vi "Add Crank Cam RTM.vi"(8 "error in (no error)":errorcluster, 11 "Node Ptr":u64 format="%.0x") -> (0 "error out":errorcluster)   [LabVIEW 2011, in "Engine Sim System Explorer.lvlib"]
uses:
  Engine Sim System Explorer.lvlib
  TypeDefs/NTeethComp.ctl
  TypeDefs/FullyCustomComp.ctl
  Shared/FullyCustomCommMode.ctl
  TypeDefs/FullyCustomProfilesComp.ctl
  <vilib>/NI Veristand/Custom Device API/Custom Device Channel.ctl
  <vilib>/NI Veristand/Custom Device API/Custom Device Channel Type.ctl
  Utility/Add Data Replay.vi
  Shared/Engine Simulation Global.vi
  <vilib>/NI Veristand/Custom Device API/Get Item Property (Variant).vi
  Utility/Set Data Replay Component Properties.vi
  <vilib>/NI Veristand/Custom Device API/NI VeriStand - Set Item Property.vi
  <vilib>/NI Veristand/Custom Device API/Set Item Property (Boolean).vi
  <vilib>/Utility/error.llb/Error Cluster From Error Code.vi
  <vilib>/NI Veristand/Custom Device API/Custom Device API.lvlib
  Engine Simulation Shared.lvlib
  <vilib>/NI Veristand/Custom Device Tools/Custom Device Utility Library/Custom Device Utility Library.lvlib
panel:
  in  "Tag":string
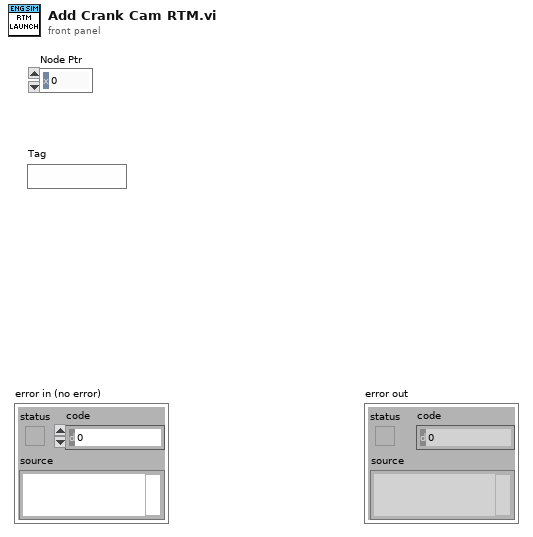
[diagram p1: front panel]
types:
  T1 = typedef "Custom Device API.lvlib/Custom Device Channel.ctl" = cluster{"Type":T2, "Units":string, "Default Value":dbl, "Faultable":bool, "Scalable":bool}
  T2 = typedef "Custom Device API.lvlib/Custom Device Channel Type.ctl" = enum16{"Input", "Output"}
  T3 = typedef "Engine Sim System Explorer.lvlib/FullyCustomComp.ctl" = cluster{"Name":string, "Comm Mode":T4, "Profiles":T5[]}
  T4 = typedef "Engine Simulation Shared.lvlib/FullyCustomCommMode.ctl" = enum16{"DMA FIFO", "FP Data Transfer"}
  T5 = typedef "Engine Sim System Explorer.lvlib/FullyCustomProfilesComp.ctl" = cluster{"Name":string, "Offset?":bool}
  T6 = typedef "Engine Sim System Explorer.lvlib/NTeethComp.ctl" = cluster{"Name":string, "TDC Offset":bool}
  T7 = typedef "Custom Device API.lvlib/Custom Device Item Ref.ctl" = u64
  T8 = typedef "Engine Sim System Explorer.lvlib/DataReplayLoopComp.ctl" = cluster{"Name":string, "DataReplays":T9[]}
  T9 = typedef "Engine Sim System Explorer.lvlib/DataReplayComp.ctl" = cluster{"Name":string, "Number":i32, "Optionals":bool[]}
  T10 = typedef "Custom Device API.lvlib/Custom Device Item Info.ctl" = cluster{"Name":string, "Is Channel":bool, "GUID":string}
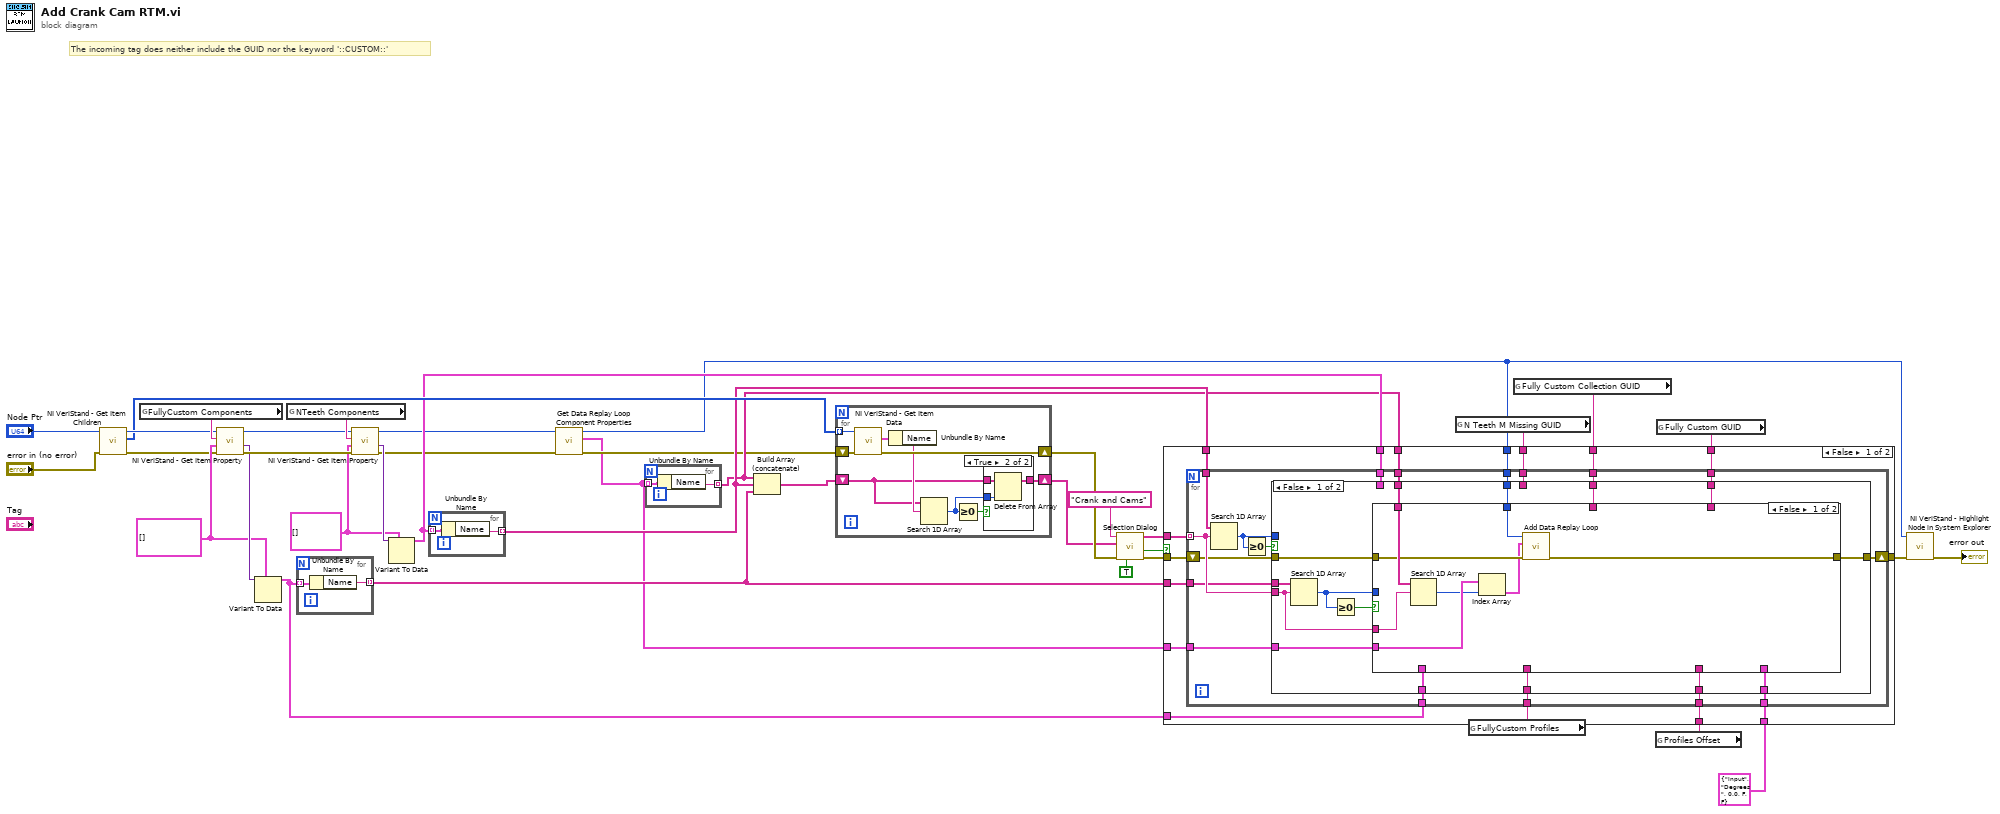
[diagram p0: block diagram]
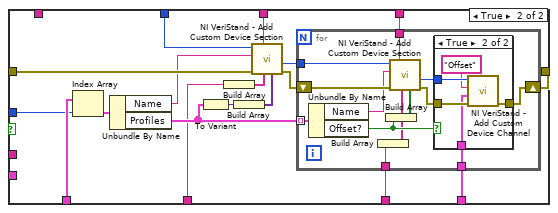
[diagram p2: hidden frame]
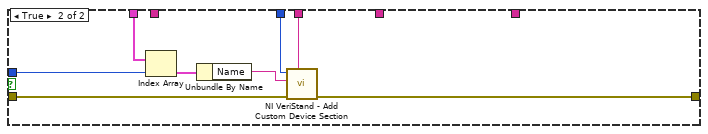
[diagram p4: hidden frame]
diagram:
  w33 = T3[] []
  w31 = T6[] []
  # "The incoming tag does neither include the GUID nor the keyword '::CUSTOM::'"
  n1 = call <vilib>:"NI VeriStand - Get Item Children.vi"("error in (no error)"="error in (no error)", "Item Ref in"="Node Ptr") -> ("error out"=w28:errorcluster, "Child Refs"=w29:T7[], "Item Ref out"=w30:T7)  [unwired: 6 in, 1 out]
  n2 = global read "Engine Simulation Global.vi" "FullyCustom Components"() -> (w38:string)
  n3 = call-poly <vilib>:"NI VeriStand - Get Item Property.vi"("error in (no error)"=w28, "Default Value"=w33, "Property Name"=w38, "Item Ref in"=w30) -> ("error out"=w35:errorcluster, "Value"=w34:variant, "Item Ref out"=w36:T7)  [unwired: 4 in, 1 out]
  n4 = Variant To Data(type=w33, Variant=w34) -> (data=w18:T3[])  [unwired: 1 in, 1 out]
  n5 = global read "Engine Simulation Global.vi" "NTeeth Components"() -> (w37:string)
  n6 = for {
    tunnel: w18 -> [w40] mode=indexing
    tunnel: [w39] -> w19 mode=indexing
    n7 = Unbundle By Name(w40) -> ("Name"=w39:string)
  }
  n8 = call-poly <vilib>:"NI VeriStand - Get Item Property.vi"("error in (no error)"=w35, "Default Value"=w31, "Property Name"=w37, "Item Ref in"=w36) -> ("error out"=w8:errorcluster, "Value"=w32:variant, "Item Ref out"=w7:T7)  [unwired: 4 in, 1 out]
  n9 = Variant To Data(type=w31, Variant=w32) -> (data=w20:T6[])  [unwired: 1 in, 1 out]
  n10 = for {
    tunnel: w20 -> [w42] mode=indexing
    tunnel: [w41] -> w21 mode=indexing
    n11 = Unbundle By Name(w42) -> ("Name"=w41:string)
  }
  n12 = call "Get Data Replay Loop Component Properties.vi"("error in (no error)"=w8, "Item Ref in"=w7) -> ("error out"=w2:errorcluster, "DataReplayLoops"=w1:T8[], "Item Ref out"=w6:T7)  [unwired: 7 in]
  n13 = for {
    tunnel: w1 -> [w44] mode=indexing
    tunnel: [w43] -> w5 mode=indexing
    n14 = Unbundle By Name(w44) -> ("Name"=w43:string)
  }
  n15 = Build Array (concatenate)(w5, w21, w19) -> (w27:string[])
  n16 = for {
    tunnel: w29 -> [w53] mode=indexing
    shift-right: [w51] -> w24
    shift-left: w2 -> [w50]
    shift-right: [w46] -> w3
    shift-left: w27 -> [w47]
    n17 = call <vilib>:"NI VeriStand - Get Item Data.vi"("error in (no error)"=w50, "Item Ref in"=w53) -> ("error out"=w51:errorcluster, "Item Info"=w52:T10)  [unwired: 6 in, 2 out]
    n18 = Unbundle By Name(w52) -> ("Name"=w48:string)
    n19 = Search 1D Array(1D array=w47, element=w48) -> (index of element=w45:i32)  [unwired: 1 in]
    n20 = Greater Or Equal To 0?(x=w45) -> (x >= 0?=w49:bool)
    n21 = case shown="True" w49 {
      tunnel: w47 -> [w54 w57]
      tunnel: [w54 w56] -> w46
      tunnel: w45 -> [_ w55]
      frame False {
      }
      frame True {
        n22 = Delete From Array(array=w57, index=w55) -> (array with subset deleted=w56:string[])  [unwired: 1 in, 1 out]
      }
    }
  }
  n23 = call "Selection Dialog.vi"("Multi-Selection?"=TRUE, "error in (no error)"=w24, "Tree Items"=w3, "Root Tag"="Crank and Cams") -> ("error out"=w22:errorcluster, "Canceled"=w4:bool, "Selected Names"=w23:string[])  [unwired: 5 in]
  n24 = global read "Engine Simulation Global.vi" "N Teeth M Missing GUID"() -> (w17:string)
  n25 = global read "Engine Simulation Global.vi" "Fully Custom Collection GUID"() -> (w16:string)
  n26 = global read "Engine Simulation Global.vi" "Profiles Offset"() -> (w9:string)
  n27 = global read "Engine Simulation Global.vi" "Fully Custom GUID"() -> (w13:string)
  n28 = case shown="False" w4 {
    tunnel: w23 -> [w73 _]
    tunnel: w22 -> [w72 w160]
    tunnel: w21 -> [w71 _]
    tunnel: w20 -> [w70 _]
    tunnel: w19 -> [w69 _]
    tunnel: w18 -> [w68 _]
    tunnel: w17 -> [w67 _]
    tunnel: w16 -> [w66 _]
    tunnel: w13 -> [w65 _]
    tunnel: T1 {"Type"=enum."Input", "Units"="Degrees", "Default Value"=0.0, "Faultable"=FALSE, "Scalable"=FALSE} ("Channel") -> [w64 _]
    tunnel: [w63 w160] -> w11
    tunnel: w9 -> [w62 _]
    tunnel: w6 -> [w60 _]
    tunnel: w5 -> [w59 _]
    tunnel: w1 -> [w58 _]
    frame False {
      n29 = global read "Engine Simulation Global.vi" "FullyCustom Profiles"() -> (w61:string)
      n30 = for {
        tunnel: w73 -> [w87] mode=indexing
        shift-right: [w84] -> w63
        shift-left: w72 -> [w83]
        tunnel: w71 -> [w91]
        tunnel: w70 -> [w90]
        tunnel: w69 -> [w86]
        tunnel: w68 -> [w85]
        tunnel: w67 -> [w82]
        tunnel: w60 -> [w81]
        tunnel: w66 -> [w80]
        tunnel: w65 -> [w79]
        tunnel: w62 -> [w78]
        tunnel: w64 -> [w77]
        tunnel: w61 -> [w76]
        tunnel: w59 -> [w75]
        tunnel: w58 -> [w74]
        n31 = Search 1D Array(1D array=w91, element=w87) -> (index of element=w88:i32)  [unwired: 1 in]
        n32 = Greater Or Equal To 0?(x=w88) -> (x >= 0?=w89:bool)
        n33 = case shown="False" w89 {
          tunnel: w90 -> [_ w159]
          tunnel: w88 -> [_ w158]
          tunnel: w87 -> [w93 _]
          tunnel: w86 -> [w106 _]
          tunnel: w85 -> [w105 _]
          tunnel: [w98 w157] -> w84
          tunnel: w83 -> [w104 w156]
          tunnel: w82 -> [_ w155]
          tunnel: w81 -> [w103 w154]
          tunnel: w80 -> [w102 _]
          tunnel: w79 -> [w101 _]
          tunnel: w78 -> [w100 _]
          tunnel: w77 -> [w99 _]
          tunnel: w76 -> [w97 _]
          tunnel: w75 -> [w94 _]
          tunnel: w74 -> [w92 _]
          frame False {
            n34 = Search 1D Array(1D array=w106, element=w93) -> (index of element=w96:i32)  [unwired: 1 in]
            n35 = Greater Or Equal To 0?(x=w96) -> (x >= 0?=w95:bool)
            n36 = case shown="False" w95 {
              tunnel: w105 -> [_ w132]
              tunnel: w104 -> [w110 w130]
              tunnel: w103 -> [w108 w129]
              tunnel: w102 -> [_ w127]
              tunnel: w101 -> [_ w120]
              tunnel: w100 -> [_ w119]
              tunnel: w99 -> [_ w118]
              tunnel: [w107 w117] -> w98
              tunnel: w97 -> [_ w116]
              tunnel: w96 -> [_ w115]
              tunnel: w94 -> [w114 _]
              tunnel: w93 -> [w113 _]
              tunnel: w92 -> [w112 _]
              frame False {
                n37 = Search 1D Array(1D array=w114, element=w113) -> (index of element=w111:i32)  [unwired: 1 in]
                n38 = Index Array(array=w112, index=w111) -> (element=w109:T8)
                n39 = call "Add Data Replay Loop.vi"("error in (no error)"=w110, "DataReplay Loop"=w109, "Crank Cams Page in"=w108) -> ("error out"=w107:errorcluster)  [unwired: 7 in, 1 out]
              }
              frame True {
                n40 = Index Array(array=w132, index=w115) -> (element=w131:T3)
                n41 = Unbundle By Name(w131) -> ("Name"=w128:string, "Profiles"=w121:T5[])
                n42 = To Variant(anything=w121) -> (Variant=w125:variant)
                n43 = Build Array(w116) -> (w124:string[])
                n44 = Build Array(w125) -> (w126:variant[])
                n45 = call <vilib>:"NI VeriStand - Add Custom Device Section.vi"("Property Values"=w126, "Property names"=w124, "GUID (Default Section)"=w127, "error in (no error)"=w130, "Section Name"=w128, "Parent Ref in"=w129) -> ("error out"=w122:errorcluster, "Section Ptr"=w123:T7)  [unwired: 2 in, 2 out]
                n46 = for {
                  tunnel: w123 -> [w145]
                  tunnel: w121 -> [w143] mode=indexing
                  tunnel: w120 -> [w141]
                  shift-right: [w136] -> w117
                  shift-left: w122 -> [w144]
                  tunnel: w119 -> [w134]
                  tunnel: w118 -> [w135]
                  n47 = Unbundle By Name(w143) -> ("Name"=w142:string, "Offset?"=w138:bool)
                  n48 = Build Array(w134) -> (w133:string[])
                  n49 = Build Array(w138) -> (w137:bool[])
                  n50 = call <vilib>:"NI VeriStand - Add Custom Device Section.vi"("Property Values"=w137, "Property names"=w133, "GUID (Default Section)"=w141, "error in (no error)"=w144, "Section Name"=w142, "Parent Ref in"=w145) -> ("error out"=w139:errorcluster, "Section Ptr"=w140:T7)  [unwired: 2 in, 2 out]
                  n51 = case shown="True" w138 {
                    tunnel: w140 -> [_ w151]
                    tunnel: w139 -> [w146 w150]
                    tunnel: [w146 w149] -> w136
                    tunnel: w135 -> [_ w148]
                    frame False {
                    }
                    frame True {
                      n52 = call <vilib>:"NI VeriStand - Add Custom Device Channel.vi"("error in (no error)"=w150, "Channel"=w148, "Channel Name"="Offset", "Parent Ref in"=w151) -> ("error out"=w149:errorcluster)  [unwired: 4 in, 3 out]
                    }
                  }
                }
              }
            }
          }
          frame True {
            n53 = Index Array(array=w159, index=w158) -> (element=w153:T6)
            n54 = Unbundle By Name(w153) -> ("Name"=w152:string)
            n55 = call <vilib>:"NI VeriStand - Add Custom Device Section.vi"("GUID (Default Section)"=w155, "error in (no error)"=w156, "Section Name"=w152, "Parent Ref in"=w154) -> ("error out"=w157:errorcluster)  [unwired: 4 in, 3 out]
          }
        }
      }
    }
    frame True {
    }
  }
  n56 = call <vilib>:"NI VeriStand - Highlight Node in System Explorer.vi"("error in (no error)"=w11, "Item Ref in"=w6) -> ("error out"=→"error out":errorcluster)  [unwired: 8 in, 1 out]
